vi "Send Write Elevator Direction.vi"(7 "Message Priority (Normal)":T2=enum."Normal", 8 "error in (no error)":errorcluster, 10 "Elevator Direction":T1, 11 "Message Enqueuer":refnum<class "Message Enqueuer.lvclass">) -> (0 "error out":errorcluster, 3 "Message Enqueuer out":refnum<class "Message Enqueuer.lvclass">)   [LabVIEW 2019, in "Simulated Display Console Actor.lvlib" / "Write Elevator Direction Msg.lvclass"]
doc: "This VI sends the message to an actor."
uses:
  Write Elevator Direction Msg.lvclass
  <vilib>/ActorFramework/Message Enqueuer/Message Enqueuer.lvclass
  C:/Program Files (x86)/National Instruments/LabVIEW 2019/vi.lib/ActorFramework/Message/Message.lvclass
  <vilib>/ActorFramework/Message Enqueuer/Message Priority.ctl
  Elevator Controller/Elevator Direction.ctl
  Elevator Controller/Sim Display Console Actor.lvclass
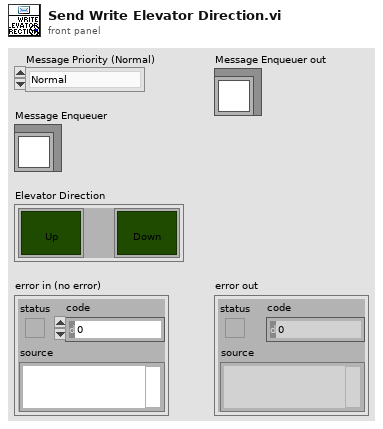
[diagram p1: front panel]
types:
  T1 = typedef "Simulated Display Console Actor.lvlib/Sim Display Console Actor.lvclass/Elevator Direction.ctl" = cluster{"Up":bool, "Down":bool}
  T2 = typedef "Actor Framework.lvlib/Message Enqueuer.lvclass/Message Priority.ctl" = enum16{"Low", "Normal", "High"}
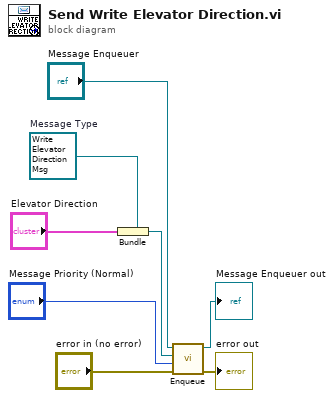
[diagram p0: block diagram]
diagram:
  w5 = refnum<class "Write Elevator Direction Msg.lvclass"> refnum  # Message Type
  n1 = Bundle(cluster=w5, "Elevator Direction") -> (w4:refnum<class "Write Elevator Direction Msg.lvclass">)
  n2 = call <vilib>:"Enqueue.vi"("error in (no error)"="error in (no error)", "Message Priority (Normal)"="Message Priority (Normal)", "Message"=w4, "Message Enqueuer in"="Message Enqueuer") -> ("error out"=→"error out":errorcluster, "Message Enqueuer out"=→"Message Enqueuer out":refnum<class "Message Enqueuer.lvclass">)  [unwired: 6 in]
